vi "Channel_Control_Read.vi"(7 "Input Channel":tag="PXI1Slot3/ai0:2", 10 "Acquisition Rate (20000)":dbl=20000.0 format="%0.2f") -> (0 "Error Out":errorcluster, 3 "READ":refnum<k21>)   [LabVIEW 2023]
uses:
  <vilib>/DAQmx/create/channels.llb/DAQmx Create Channel (AI-Voltage-Basic).vi
  <vilib>/DAQmx/configure/timing.llb/DAQmx Timing (Sample Clock).vi
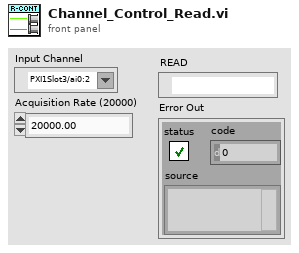
[diagram p1: front panel]
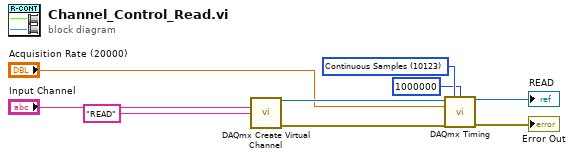
[diagram p0: block diagram]
diagram:
  w2 = 10123 items=["Finite Samples"=10178, "Continuous Samples"=10123, "Hardware Timed Single Point"=12522] ("sample mode")
  n1 = call-poly <vilib>:"DAQmx Create Virtual Channel.vi"("physical channels"="Input Channel", "name to assign"="READ") -> ("task out"=w8:refnum<k21>, "error out"=w6:errorcluster)  [unwired: 12 in]
  n2 = call-poly <vilib>:"DAQmx Timing.vi"("task/channels in"=w8, "sample mode"=w2, "samples per channel"=1000000, "rate"="Acquisition Rate (20000)", "error in"=w6) -> ("task out"=→"READ":refnum<k21>, "error out"=→"Error Out":errorcluster)  [unwired: 9 in]
